vi "SMC_Stop.vi"(8 "error in (no error)":errorcluster) -> (0 "error out":errorcluster)   [LabVIEW 2015]
uses:
  SMC_SubVIs.llb/SMC_ManagerMode.ctl
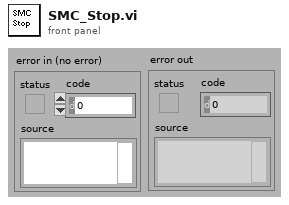
[diagram p1: front panel]
types:
  T1 = typedef "SMC_ManagerMode.ctl" = enum16{"Init", "Get", "SetPosition", "SetStatus", "SetMoving", "SetControllerNr"}
  T2 = typedef "SMC Paras.ctl" = cluster{"VENUS Language":T3, "Number of Axis":u8, "Controller Nr":u8, "Simulation":bool}
  T3 = typedef "VENUSNr.ctl" = enum16{"VENUS 2", "VENUS 1"}
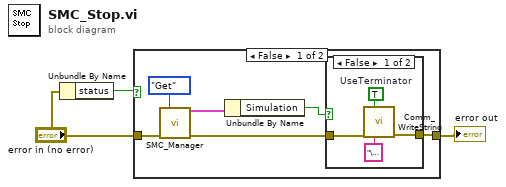
[diagram p0: block diagram]
diagram:
  n1 = Unbundle By Name("error in (no error)") -> ("status"=w3:bool)
  n2 = case shown="False" w3 {
    tunnel: "error in (no error)" -> [w8 w15]
    tunnel: [w6 w15] -> w1
    frame False {
      n3 = call "SMC_Manager.vi"("Mode"=SMC_ManagerMode."Get", "error in (no error)"=w8) -> ("SMC Parameter Out"=w5:T2, "error out"=w7:errorcluster)  [unwired: 9 in, 3 out]
      n4 = Unbundle By Name(w5) -> ("Simulation"=w4:bool)
      n5 = case shown="False" w4 {
        tunnel: w7 -> [w12 w14]
        tunnel: [w11 w14] -> w6
        frame False {
          w10 = TRUE  # UseTerminator
          n6 = call "Comm_WriteString.vi"("string to write"="\u0003" ("Substring"), "error in (no error)"=w12, "UseTerminator"=w10) -> ("error out"=w11:errorcluster)  [unwired: 8 in]
        }
        frame True {
          # "Simulation"
        }
      }
    }
    frame True {
      # "Error, do nothing"
    }
  }
  "error out" <- w1
